vi "Send to Client.vi"(6 "Timeout ms (1000)":i32=1000, 7 "Format (Text)":T1, 8 "error in (no error)":errorcluster, 9 "Payload":string, 10 "Client URI String":string, 11 "Basic WebSocket Manager in":refnum<class "Basic WebSocket Manager.lvclass">) -> (0 "error out":errorcluster, 3 "Basic WebSocket Manager out":refnum<class "Basic WebSocket Manager.lvclass">)   [LabVIEW 2020, in "HTTP Server.lvlib" / "Basic WebSocket Manager.lvclass"]
uses:
  Basic WebSocket Manager.lvclass
  Basic WebSocket Manager.lvclass/Basic WebSocket Manager.ctl
  WebSocket Client/WebSocket Client.lvclass
  WebSocket Format.ctl
  HTTP Server.lvlib
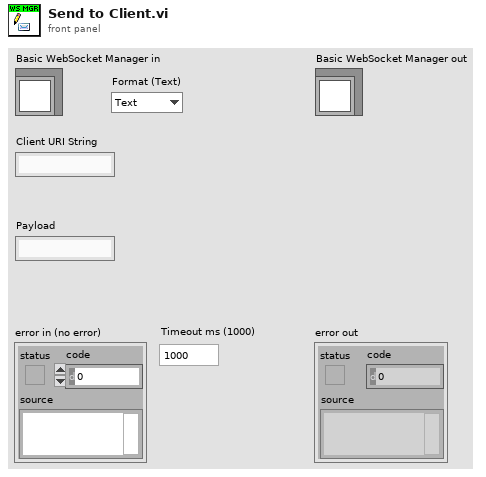
[diagram p1: front panel]
types:
  T1 = typedef "HTTP Server.lvlib/WebSocket Format.ctl" = enum16{"Text", "Binary"}
  T2 = typedef "HTTP Server.lvlib/Basic WebSocket Manager.lvclass/Ref Data.ctl" = cluster{"Clients":map{string, refnum<class "WebSocket Client.lvclass">}}
  T3 = map{string, refnum<class "WebSocket Client.lvclass">}
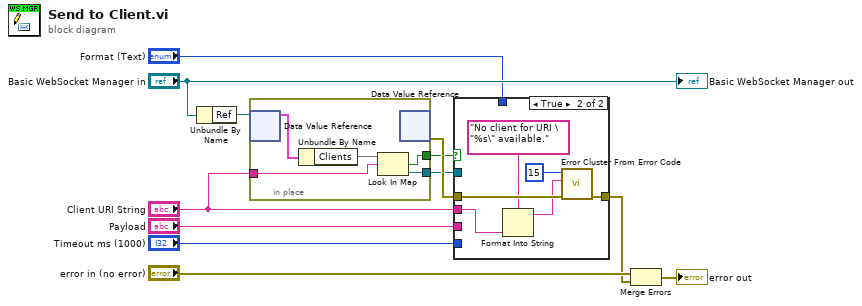
[diagram p0: block diagram]
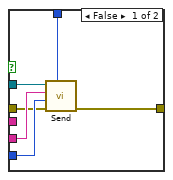
[diagram p2: hidden frame]
diagram:
  n1 = Unbundle By Name("Basic WebSocket Manager in") -> ("Ref"=w10:refnum<data-value>)
  n2 = in-place {
    in-place-border: "Client URI String" -> [w15]
    in-place-border: [w14] -> w7
    in-place-border: [w13] -> w8
    n3 = in-place-dvr #1(w10) -> (w17:T2)  [unwired: 1 out]
    n4 = Unbundle By Name(w17) -> ("Clients"=w16:T3)
    n5 = Look In Map(map=w16, key=w15) -> (key not found?=w13:bool, value=w14:refnum<class "WebSocket Client.lvclass">)  [unwired: 1 in]
    n6 = in-place-dvr #1() -> (w12:errorcluster)  [unwired: 1 in, 1 out]
  }
  n7 = case shown="True" w8 {
    tunnel: w7 -> [w23 _]
    tunnel: "Format (Text)" -> [w22 _]
    tunnel: "Payload" -> [w21 _]
    tunnel: "Timeout ms (1000)" -> [w20 _]
    tunnel: [w19 w28] -> w1
    tunnel: w12 -> [w18 w29]
    tunnel: "Client URI String" -> [_ w27]
    frame False {
      n8 = call "Send.vi"("Format (Text)"=w22, "error in (no error)"=w18, "Timeout ms (1000)"=w20, "Payload"=w21, "WebSocket Client in"=w23) -> ("error out"=w19:errorcluster)  [unwired: 5 in, 1 out]
    }
    frame True {
      n9 = Format Into String(format string="No client for URI \"%s\" available.", w27) -> (resulting string=w25:string)  [unwired: 2 in, 1 out]
      n10 = call <vilib>:"Error Cluster From Error Code.vi"("error in (no error)"=w29, "error message (\"\")"=w25, "error code (0)"=15) -> ("error out"=w28:errorcluster)  [unwired: 6 in]
    }
  }
  n11 = Merge Errors("error in (no error)", w1) -> (→"error out":errorcluster)
  "Basic WebSocket Manager out" <- "Basic WebSocket Manager in"
